vi "increment_global_var.vi"() -> ()   [LabVIEW 2025]
panel:
  in  "Numeric":dbl
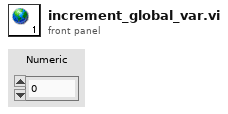
[diagram p1: front panel]
diagram:
